vi "find_PlotObject_by_Name.vi"(10 "Plot Name/ID":string, 11 "PlotObj Array in":refnum<class "Plots.lvclass">[](array[class])) -> (0 "index of Object in Array":i32, 1 "found?":bool, 2 "found PlotObj out":refnum<class "Plots.lvclass">, 3 "PlotObj Array out":refnum<class "Plots.lvclass">[](array[class]))   [LabVIEW 2017]
doc: "Find the correct PlotObject by the Name/ID of the Plot"
uses:
  Classes/Plots/Plots.lvclass
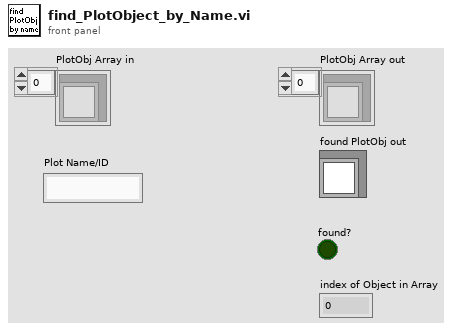
[diagram p1: front panel]
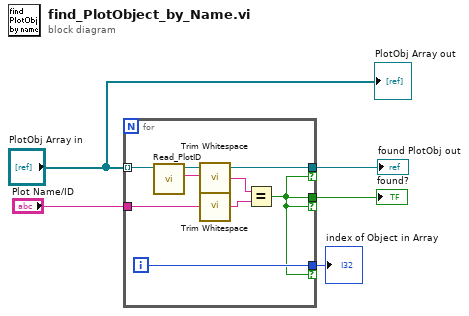
[diagram p0: block diagram]
diagram:
  n1 = for {
    tunnel: "Plot Name/ID" -> [w13]
    tunnel: [w10] -> w4 if=w6
    tunnel: "PlotObj Array in" -> [w8] mode=indexing
    tunnel: [w6] -> w3 if=w6
    tunnel: [w7] -> w1 if=w6
    i -> [w7]
    n2 = call-dynamic "Read_PlotID.vi"("Plots in"=w8) -> ("PlotID"=w9:string, "Plots out"=w10:refnum<class "Plots.lvclass">)  [unwired: 8 in, 1 out]
    n3 = call <vilib>:"Trim Whitespace.vi"("string"=w9) -> ("trimmed string"=w12:string)  [unwired: 1 in]
    n4 = call <vilib>:"Trim Whitespace.vi"("string"=w13) -> ("trimmed string"=w11:string)  [unwired: 1 in]
    n5 = Equal?(x=w12, y=w11) -> (x = y?=w6:bool)
  }
  "found PlotObj out" <- w4
  "found?" <- w3
  "index of Object in Array" <- w1
  "PlotObj Array out" <- "PlotObj Array in"
